vi "user.me.vi"(8 "error in":errorcluster, 11 "Client in":refnum<class "Client.lvclass">) -> (0 "error out":errorcluster, 2 "User":refnum<class "User.lvclass">, 3 "Client out":refnum<class "Client.lvclass">)   [LabVIEW 2020, in "Client.lvclass"]
doc: "Returns a handle to the currently authenticated user."
uses:
  Client.lvclass
  Client.lvclass/Client.ctl
  client.lvlib
  User/User.lvclass
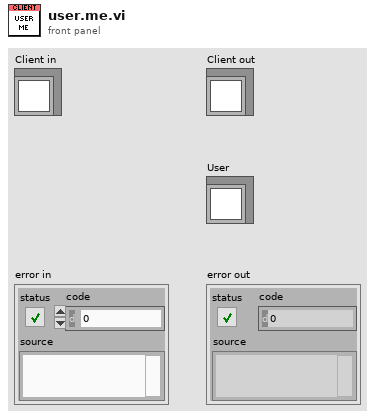
[diagram p1: front panel]
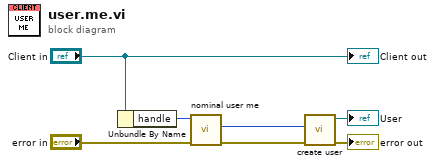
[diagram p0: block diagram]
diagram:
  n1 = Unbundle By Name("Client in") -> ("handle"=w6:i32)
  n2 = call "nominal user me.vi"("error in (no error)"="error in", "client"=w6) -> ("error out"=w1:errorcluster, "out_user out"=w4:i32)  [unwired: 7 in, 1 out]
  n3 = call "create user.vi"("error in (no error)"=w1, "handle"=w4) -> ("error out"=→"error out":errorcluster, "User out"=→"User":refnum<class "User.lvclass">)  [unwired: 8 in]
  "Client out" <- "Client in"
